vi "Get Point by key.vi"(8 "error in (no error)":errorcluster caption="错误输入（无错误）", 10 "Key":string, 11 "Dictionary In":refnum<class "Dictionary.lvclass"> caption="DNL_LabVIEW Object in") -> (0 "error out":errorcluster caption="错误输出", 1 "Key Exist?":bool, 2 "point":cluster{"x":i16, "y":i16} caption="点", 3 "Dictionary Out":refnum<class "Dictionary.lvclass"> caption="DNL_LabVIEW Object out")   [LabVIEW 2012, in "Dictionary.lvclass"]
uses:
  Dictionary.lvclass
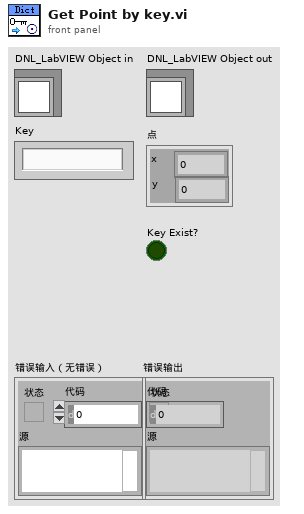
[diagram p1: front panel]
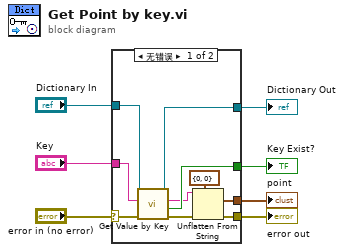
[diagram p0: block diagram]
diagram:
  n1 = case shown="无错误" "error in (no error)" {
    selector: "error in (no error)" -> [w15 w19]
    tunnel: [w11 w19] -> w6
    tunnel: [w16 w18] -> w4
    tunnel: "Dictionary In" -> [w17 w18]
    tunnel: [w14 _] -> w3
    tunnel: [w9 _] -> w2
    tunnel: "Key" -> [w8 _]
    frame No Error {
      n2 = call "Get Value by Key.vi"("error in (no error)"=w15, "Key"=w8, "Dictionary In"=w17) -> ("error out"=w12:errorcluster, "Key Exist?"=w14:bool, "Value"=w13:string, "Dictionary Out"=w16:refnum<class "Dictionary.lvclass">)  [unwired: 5 in]
      n3 = Unflatten From String(type=cluster{"x":i16, "y":i16} {"x"=0, "y"=0} ("point"), binary string=w13, error in (no error)=w12) -> (value=w9:cluster{"x":i16, "y":i16}, error out=w11:errorcluster)  [unwired: 2 in, 1 out]
    }
    frame Error {
    }
  }
  "error out" <- w6
  "Dictionary Out" <- w4
  "point" <- w2
  "Key Exist?" <- w3
